vi "Find Parse State Queue from While Loop.vi"(8 "error in (no error)":errorcluster, 11 "WhileLoop in":refnum<vi>) -> (0 "error out":errorcluster, 1 "CaseStructure":refnum<vi>, 2 "Parse State Queue":refnum<vi>, 3 "WhileLoop out":refnum<vi>)   [LabVIEW 2017, in "csmHelper-Relationship.lvlib"]
doc: "-- <b>输入控件</b> --\n- <b>error in (no error)</b>:\n- <B>error in</B> can accept error information wired from VIs previously called. Use this information to decide if any functionality should be bypassed in the event of errors from other VIs.\n\nRight-click the <B>error in</B> control on the front panel and select <B>Explain Error</B> or <B>Explain Warning</B> from the shortcut menu for more information about the error.\n- <b>WhileLoop in</b>:\n\n\n-- <b>输出控件</b> --\n- <b>error out</b>:\n- <B>error in</B> can accept error information wired from VIs previously called. Use this information to decide if any functionality should be bypassed in the event of errors from other VIs.\n\nRight-click the <B>error in</B> control on the front panel and select <B>Explain Error</B> or <B>Explain Warning</B> from the shortcut menu for more information about the error.\n- <b>CaseStructure</b>:\n\n- <b>Parse State Queue</b>:\n\n- <b>WhileLoop out</b>:"
uses:
  csmHelper-Relationship.lvlib
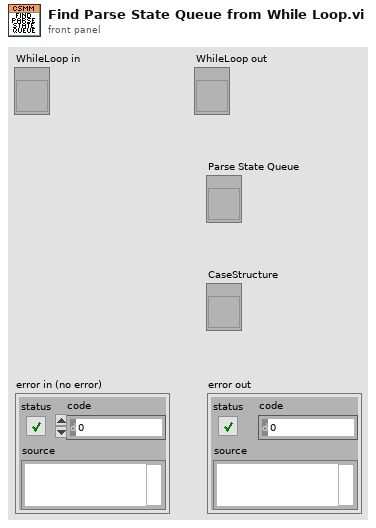
[diagram p1: front panel]
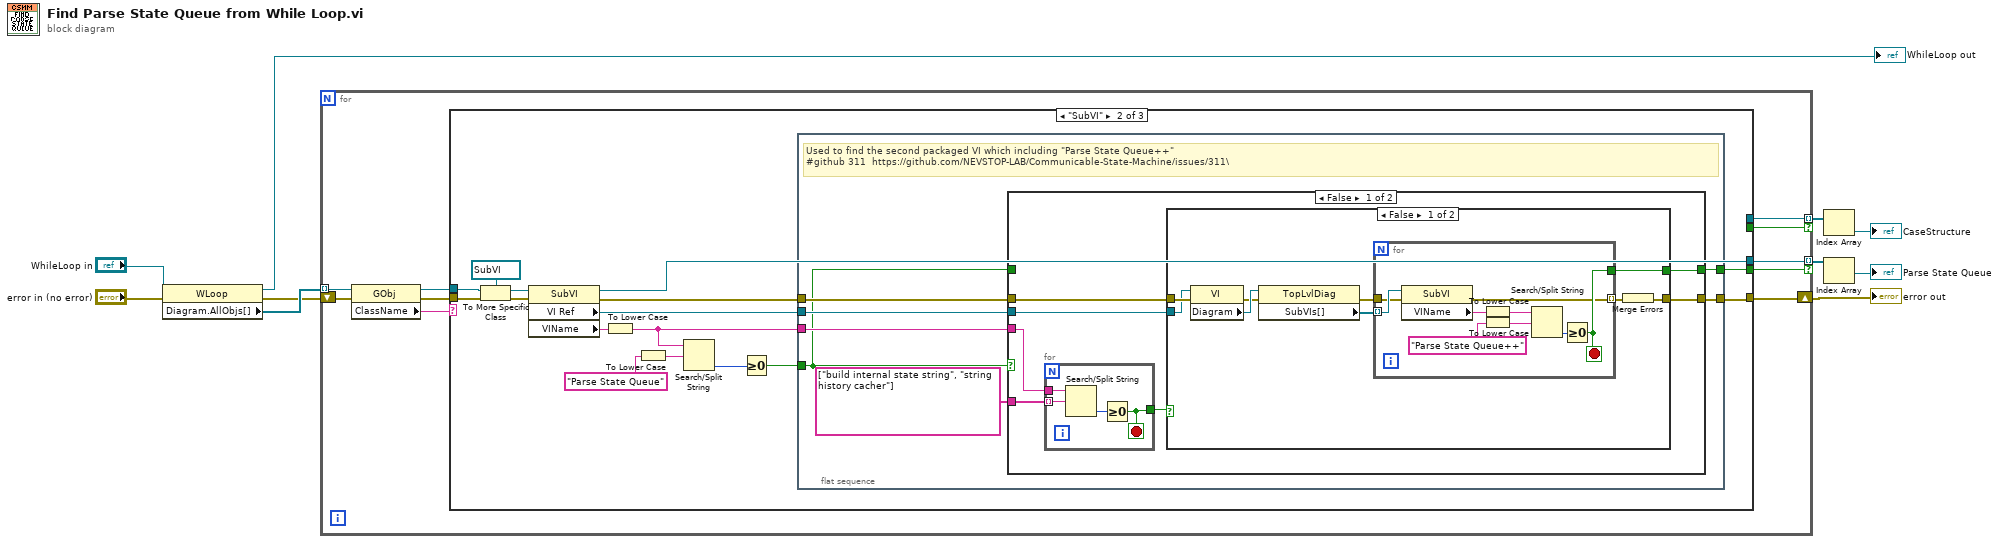
[diagram p0: block diagram]
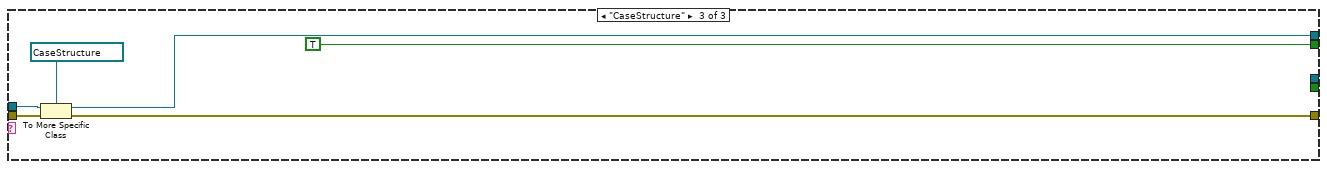
[diagram p5: hidden frame]
diagram:
  n1 = property on="Property Node" class="WLoop"(reference="WhileLoop in", error in="error in (no error)") -> (reference out=→"WhileLoop out":refnum<vi>, error out=w7:errorcluster, "Diagram.AllObjs[]"=w10:refnum<vi>[])
  n2 = for {
    tunnel: w10 -> [w20] mode=indexing
    shift-right: [w15] -> w6
    shift-left: w7 -> [w16]
    tunnel: [w14] -> w3 mode=indexing if=w11
    tunnel: [w13] -> w5 mode=indexing if=w12
    n3 = property class="GObj"(reference=w20, error in=w16) -> (reference out=w18:refnum<vi>, error out=w17:errorcluster, "ClassName"=w19:string)
    n4 = case shown="\"SubVI\"" w19 {
      tunnel: w18 -> [_ w36 w81]
      tunnel: w17 -> [w21 w35 w80]
      tunnel: [w21 w26 w79] -> w15
      tunnel: [_ w31 _] -> w14
      tunnel: [_ _ w78] -> w13
      tunnel: [_ _ TRUE] -> w12
      tunnel: [_ w27 _] -> w11
      frame Default {
      }
      frame "SubVI" {
        n5 = To More Specific Class(target class=refnum<vi> refnum ("SubVI Refnum"), reference=w36, error in=w35) -> (specific class reference=w34:refnum<vi>, error out=w33:errorcluster)
        n6 = property class="SubVI"(reference=w34, error in=w33) -> (reference out=w31:refnum<vi>, error out=w28:errorcluster, "VI Ref"=w24:refnum<vi>, "VIName"=w25:string)
        n7 = To Lower Case(string=w25) -> (all lower case string=w22:string)
        n8 = To Lower Case(string="Parse State Queue" ("VI Name")) -> (all lower case string=w30:string)
        n9 = Search/Split String(string=w22, search string/char (-)=w30) -> (offset of match=w29:i32)  [unwired: 1 in, 2 out]
        n10 = Greater Or Equal To 0?(x=w29) -> (x >= 0?=w23:bool)
        n11 = flat-sequence {
          tunnel: w28 -> [w44]
          tunnel: [w43] -> w26
          tunnel: w22 -> [w42]
          tunnel: [w41] -> w27
          tunnel: w24 -> [w40]
          tunnel: w23 -> [w38]
          frame #0 {
            # "Used to find the second packaged VI which including \"Parse State Queue++\"\n#github 311  https://github.com/NEVSTOP-LAB/Communicable-State-Machine/issues/311\\"
            n12 = case shown="False" w38 {
              tunnel: w44 -> [w49 w76]
              tunnel: [w48 w76] -> w43
              tunnel: w42 -> [w50 _]
              tunnel: string[] ["build internal state string", "string history cacher"] ("all lower case string") -> [w51 _]
              tunnel: [w46 w75] -> w41
              tunnel: w38 -> [_ w75]
              tunnel: w40 -> [w47 _]
              frame False {
                n13 = for {
                  tunnel: w51 -> [w54] mode=indexing
                  tunnel: w50 -> [w55]
                  tunnel: [w52] -> w45
                  stop <- w52 stop-if-true
                  n14 = Search/Split String(string=w55, search string/char (-)=w54) -> (offset of match=w53:i32)  [unwired: 1 in, 2 out]
                  n15 = Greater Or Equal To 0?(x=w53) -> (x >= 0?=w52:bool)
                }
                n16 = case shown="False" w45 {
                  tunnel: w49 -> [w59 w74]
                  tunnel: [w63 w74] -> w48
                  tunnel: w47 -> [w58 _]
                  tunnel: [w56 _] -> w46
                  frame False {
                    n17 = property class="VI"(reference=w58, error in=w59) -> (error out=w61:errorcluster, "Diagram"=w62:refnum<vi>)  [unwired: 1 out]
                    n18 = property class="TopLvlDiag"(reference=w62, error in=w61) -> (error out=w60:errorcluster, "SubVIs[]"=w57:refnum<vi>[])  [unwired: 1 out]
                    n19 = for {
                      tunnel: w57 -> [w73] mode=indexing
                      tunnel: w60 -> [w72]
                      tunnel: [w66] -> w56
                      tunnel: [w65] -> w64 mode=indexing
                      stop <- w66 stop-if-true
                      n20 = property class="SubVI"(reference=w73, error in=w72) -> (error out=w65:errorcluster, "VIName"=w71:string)  [unwired: 1 out]
                      n21 = To Lower Case(string=w71) -> (all lower case string=w69:string)
                      n22 = To Lower Case(string="Parse State Queue++" ("VI Name")) -> (all lower case string=w67:string)
                      n23 = Search/Split String(string=w69, search string/char (-)=w67) -> (offset of match=w70:i32)  [unwired: 1 in, 2 out]
                      n24 = Greater Or Equal To 0?(x=w70) -> (x >= 0?=w66:bool)
                    }
                    n25 = Merge Errors(w64) -> (w63:errorcluster)
                  }
                  frame True {
                  }
                }
              }
              frame True {
              }
            }
          }
        }
      }
      frame "CaseStructure" {
        n26 = To More Specific Class(target class=refnum<vi> refnum ("CaseSel Refnum"), reference=w81, error in=w80) -> (specific class reference=w78:refnum<vi>, error out=w79:errorcluster)
      }
    }
  }
  "error out" <- w6
  n27 = Index Array(array=w5) -> (element=→"CaseStructure":refnum<vi>)  [unwired: 1 in]
  n28 = Index Array(array=w3) -> (element=→"Parse State Queue":refnum<vi>)  [unwired: 1 in]
